vi "y cut plot.vi"(4 "YScale.Multiplier":dbl, 6 "YScale.Offset":dbl, 7 "Intensity V vs I and B":dbl[][](array[numeric]), 9 "XScale.Multiplier":dbl, 10 "XScale.Offset":dbl, 11 "Cursor.Cursor X":dbl) -> (3 "Cluster":cluster{dbl[], "Intensity V vs I and B":dbl[]})   [LabVIEW 2021]
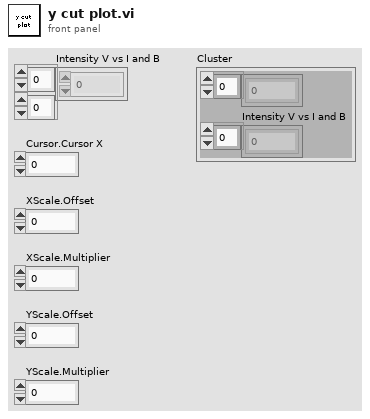
[diagram p1: front panel]
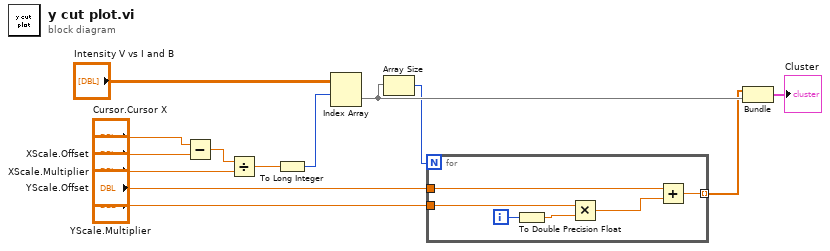
[diagram p0: block diagram]
diagram:
  n1 = Subtract(x="Cursor.Cursor X", y="XScale.Offset") -> (x-y=w3:dbl)
  n2 = Divide(x=w3, y="XScale.Multiplier") -> (x/y=w6:dbl)
  n3 = To Long Integer(number=w6) -> (32bit integer=w7:i32)
  n4 = Index Array(array="Intensity V vs I and B", index (row)=w7) -> (element=w12:dbl[])  [unwired: 1 in]
  n5 = Array Size(array=w12) -> (size(s)=w8:i32)
  n6 = for {
    N: w8 -> [_]
    tunnel: "YScale.Multiplier" -> [w18]
    tunnel: "YScale.Offset" -> [w15]
    tunnel: [w14] -> w11 mode=indexing
    i -> [w19]
    n7 = To Double Precision Float(number=w19) -> (double precision float=w17:dbl)
    n8 = Multiply(x=w18, y=w17) -> (x*y=w16:dbl)
    n9 = Add(x=w15, y=w16) -> (x+y=w14:dbl)
  }
  n10 = Bundle(w11, "Intensity V vs I and B"=w12) -> (→"Cluster":cluster{dbl[], "Intensity V vs I and B":dbl[]})  [unwired: 1 in]
